vi "Actividad Extra 14 (2).vi"() -> ()   [LabVIEW 2018]
panel:
  out "Numeric 2":i32
  out "Pos Enemigos":i32
  out "Estado Actual":string
  out "Vidas Restantes":i32
  out "element 2":bool
  out "element 1":bool
  out "Posicion de la Nave":bool
  out "2":bool
  out "1":bool
  out "0":bool
  out "Disparos Restantes":i32
  out "Turno (5s)":i32 caption="Elapsed Time (s)"
  out "Nave Dispara Laser":bool
  in  "Disparar Laser":bool
  out "Nave Vuela a la Derecha":bool
  out "Nave Vuela a la Izq":bool
  in  "Izquierda":bool
  in  "Derecha":bool
  in  "ME RINDO":bool
  out "Jugador":bool[](array[boolean])
  out "Enemigos":bool[][](array[boolean])
  # "JUEGO NAVE ESPACIAL"
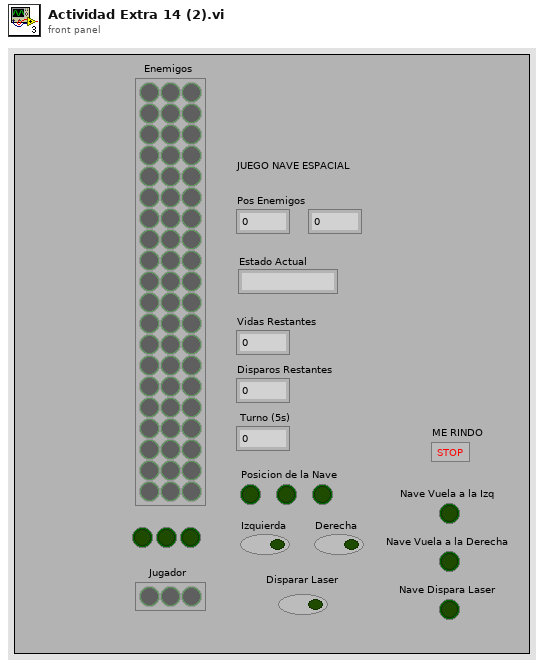
[diagram p1: front panel]
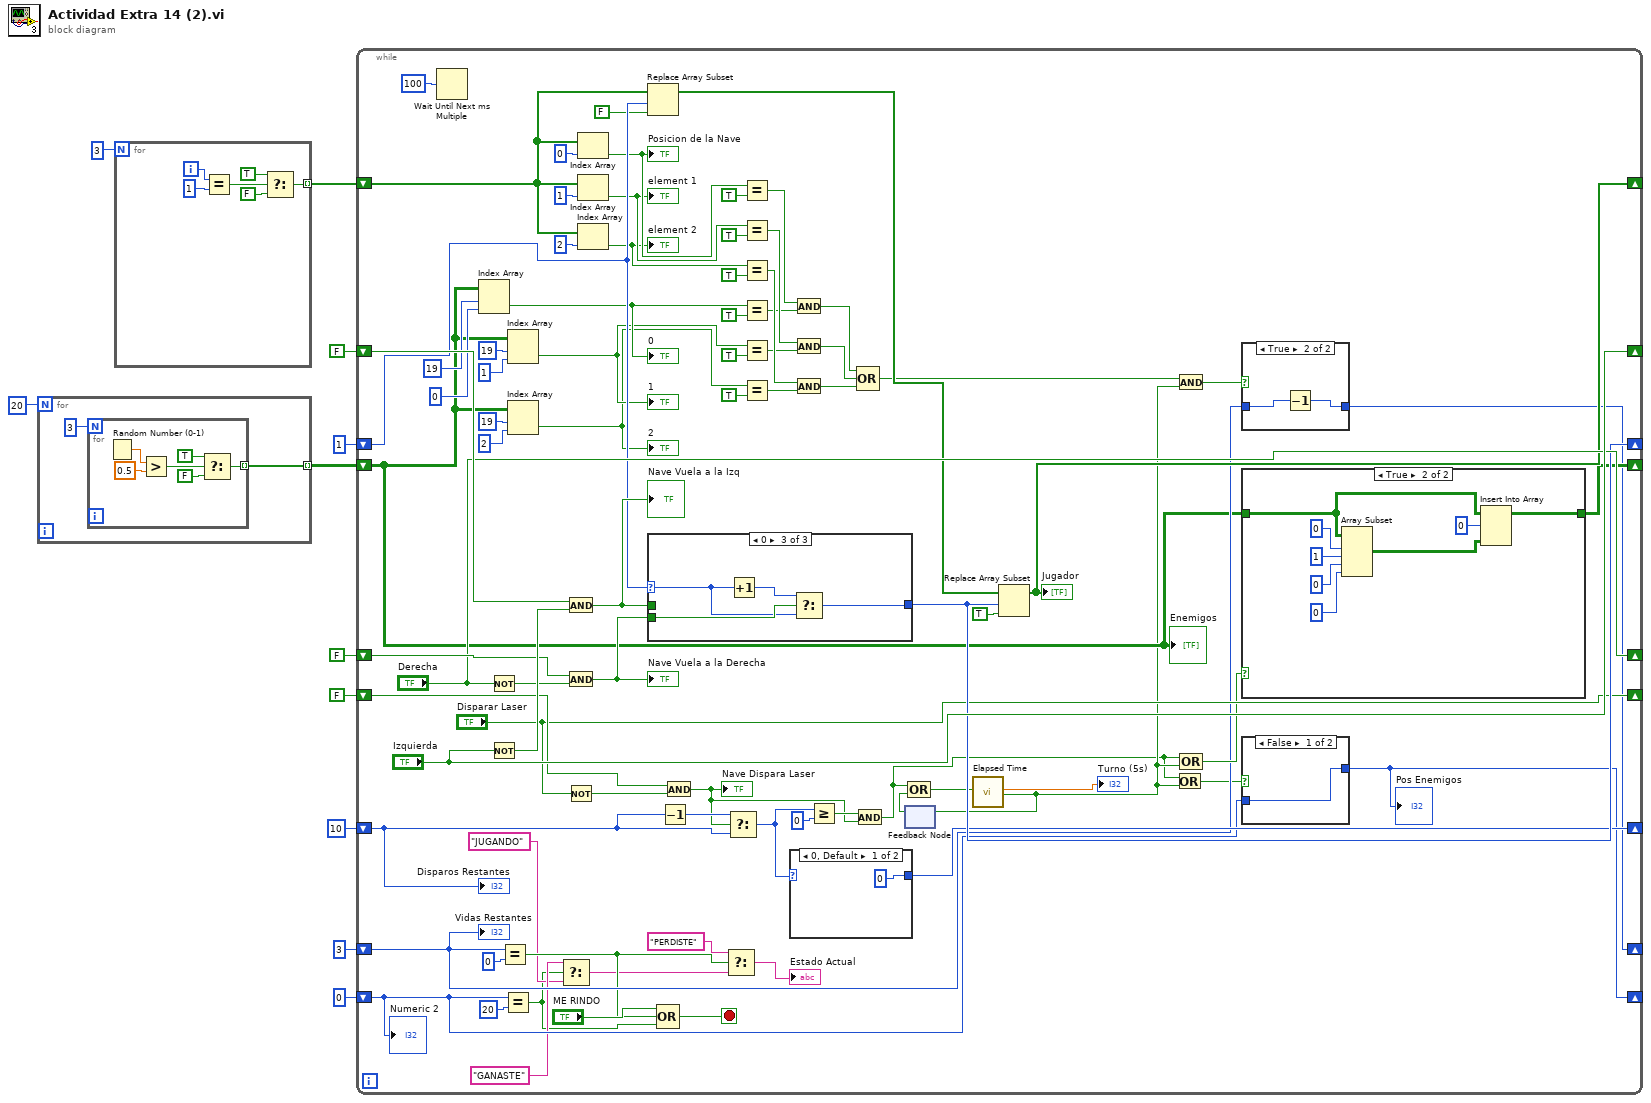
[diagram p0: block diagram]
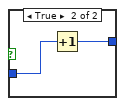
[diagram p2: hidden frame]
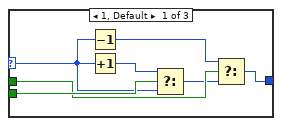
[diagram p6: hidden frame]
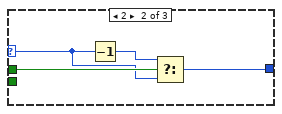
[diagram p7: hidden frame]
diagram:
  n1 = for {
    N: 20 -> [_]
    tunnel: [w12] -> w9 mode=indexing
    n2 = for {
      N: 3 -> [_]
      tunnel: [w14] -> w12 mode=indexing
      n3 = Random Number (0-1)() -> (number: 0 to 1=w19:dbl)
      n4 = Greater?(x=w19, y=0.5) -> (0:w17:bool)
      n5 = Select(t=TRUE, s=w17, f=FALSE) -> (s? t:f=w14:bool)
    }
  }
  n6 = for {
    N: 3 -> [_]
    tunnel: [w20] -> w8 mode=indexing
    i -> [w25]
    n7 = Equal?(x=w25, y=1) -> (x = y?=w23:bool)
    n8 = Select(t=TRUE, s=w23, f=FALSE) -> (s? t:f=w20:bool)
  }
  n9 = while {
    shift-right: [w93] -> _
    shift-left: w8 -> [w72]
    shift-right: [w89] -> _
    shift-left: w9 -> [w37]
    shift-right: ["Izquierda"] -> _
    shift-left: FALSE -> [w106]
    shift-right: ["Derecha"] -> _
    shift-left: FALSE -> [w103]
    shift-right: [w98] -> _
    shift-left: 1 -> [w97]
    shift-right: ["Disparar Laser"] -> _
    shift-left: FALSE -> [w92]
    shift-right: [w79] -> _
    shift-left: 10 -> [w84]
    shift-right: [w68] -> _
    shift-left: 3 -> [w67]
    shift-right: [w35] -> _
    shift-left: 0 -> [w31]
    stop <- w64 stop-if-true
    n10 = Wait Until Next ms Multiple(millisecond multiple=u32 100) -> ()  [unwired: 1 out]
    n11 = Index Array "Index Array"(array=w37, index (row)=19, index (col)=0 ("disabled index (col)")) -> (element=w44:bool)
    "0" <- w44
    n12 = Not(x="Derecha") -> (.not. x?=w102:bool)
    n13 = Not(x="Izquierda") -> (.not. x?=w105:bool)
    n14 = Equal?(x=w67, y=0) -> (x = y?=w40:bool)
    n15 = Equal?(x=w31, y=20) -> (x = y?=w26:bool)
    n16 = Index Array(array=w37, index (row)=19, index (col)=1 ("disabled index (col)")) -> (element=w43:bool)
    "1" <- w43
    n17 = Index Array(array=w37, index (row)=19, index (col)=2 ("disabled index (col)")) -> (element=w42:bool)
    "2" <- w42
    n18 = Select(t="GANASTE" ("f"), s=w26, f="JUGANDO") -> (s? t:f=w29:string)
    n19 = And(x=w106, y=w105) -> (x .and. y?=w99:bool)
    "Nave Vuela a la Izq" <- w99
    n20 = And(x=w103, y=w102) -> (x .and. y?=w100:bool)
    "Nave Vuela a la Derecha" <- w100
    n21 = Not(x="Disparar Laser") -> (.not. x?=w91:bool)
    n22 = Index Array(array=w72, index=0) -> (element=w62:bool)
    "Posicion de la Nave" <- w62
    n23 = Index Array(array=w72, index=1) -> (element=w60:bool)
    "element 1" <- w60
    n24 = Index Array(array=w72, index=2) -> (element=w57:bool)
    "element 2" <- w57
    n25 = Replace Array Subset "Replace Array Subset"(array=w72, new element=FALSE ("new element/subarray"), index=w97) -> (w95:bool[])
    n26 = case shown="0" w97 {
      selector: w97 -> [w127 w133 w136]
      tunnel: w100 -> [w131 _ w139]
      tunnel: [w125 w132 w137] -> w98
      tunnel: w99 -> [w129 w135 _]
      frame 1, Default {
        n27 = Decrement(x=w127) -> (x-1=w128:i32)
        n28 = Increment(x=w127) -> (x+1=w130:i32)
        n29 = Select(t=w130, s=w131, f=w127) -> (s? t:f=w126:i32)
        n30 = Select(t=w128, s=w129, f=w126) -> (s? t:f=w125:i32)
      }
      frame 2 {
        n31 = Decrement(x=w133) -> (x-1=w134:i32)
        n32 = Select(t=w134, s=w135, f=w133) -> (s? t:f=w132:i32)
      }
      frame 0 {
        n33 = Increment(x=w136) -> (x+1=w138:i32)
        n34 = Select(t=w138, s=w139, f=w136) -> (s? t:f=w137:i32)
      }
    }
    n35 = Compound Arithmetic op=OR("ME RINDO", w40, w26) -> (w64:bool)
    n36 = Decrement(x=w84) -> (x-1=w83:i32)
    n37 = And(x=w92, y=w91) -> (x .and. y?=w33:bool)
    "Nave Dispara Laser" <- w33
    n38 = Select(t="PERDISTE", s=w40, f=w29) -> (s? t:f=→"Estado Actual":string)
    n39 = Select(t=w83, s=w33, f=w84) -> (s? t:f=w80:i32)
    n40 = Equal?(x=w62, y=TRUE) -> (x = y?=w56:bool)
    n41 = Equal?(x=w60, y=TRUE) -> (x = y?=w55:bool)
    n42 = Equal?(x=w57, y=TRUE) -> (x = y?=w54:bool)
    n43 = Equal?(x=w44, y=TRUE) -> (x = y?=w48:bool)
    n44 = Equal?(x=w43, y=TRUE) -> (x = y?=w50:bool)
    n45 = Equal?(x=w42, y=TRUE) -> (x = y?=w49:bool)
    n46 = case shown="0, Default" w80 {
      selector: w80 -> [_ w115]
      tunnel: [0 w115] -> w79
      frame 0, Default {
      }
      frame 1.. {
      }
    }
    n47 = And(x=w56, y=w48) -> (x .and. y?=w47:bool)
    n48 = And(x=w55, y=w50) -> (x .and. y?=w46:bool)
    n49 = And(x=w54, y=w49) -> (x .and. y?=w45:bool)
    n50 = Greater Or Equal?(x=w80, y=0) -> (x >= y?=w81:bool)
    n51 = And(x=w81, y=w33) -> (x .and. y?=w30:bool)
    n52 = Compound Arithmetic op=OR(w47, w46, w45) -> (w41:bool)
    n53 = feedback #1() -> (w86:bool)  [unwired: 1 in]
    n54 = Compound Arithmetic op=OR(w30, w86) -> (w87:bool)
    n55 = call "Elapsed Time"("Reset"=w87) -> ("Elapsed Time (s)"=→"Turno (5s)":dbl, "Time has Elapsed"=w32:bool)  [unwired: 11 in, 6 out]
    n56 = feedback-in #1(w32) -> ()
    n57 = Replace Array Subset(array=w95, new element=TRUE ("new element/subarray"), index=w98) -> (w93:bool[])
    "Jugador" <- w93
    n58 = Or(x=w30, y=w32) -> (x .or. y?=w36:bool)
    n59 = And(x=w41, y=w32) -> (x .and. y?=w63:bool)
    n60 = Compound Arithmetic op=OR(w30, w32) -> (w85:bool)
    n61 = case shown="True" w63 {
      tunnel: w67 -> [w111 w113]
      tunnel: [w111 w112] -> w68
      frame False {
      }
      frame True {
        n62 = Decrement(x=w113) -> (x-1=w112:i32)
      }
    }
    n63 = case shown="True" w85 {
      tunnel: w37 -> [w116 w120]
      tunnel: [w116 w117] -> w89
      frame False {
      }
      frame True {
        n64 = Array Subset "Array Subset"(array=w120, index (row)=0 ("index"), length (row)=1 ("length"), index (col)=0 ("index"), length (col)=0 ("length")) -> (w119:bool[][])
        n65 = Insert Into Array "Insert Into Array"(array=w120, index (row)=0, new element=w119) -> (w117:bool[][])  [unwired: 1 in]
      }
    }
    n66 = case shown="False" w36 {
      tunnel: w31 -> [w108 w110]
      tunnel: [w108 w109] -> w35
      frame False {
      }
      frame True {
        n67 = Increment(x=w110) -> (x+1=w109:i32)
      }
    }
    "Pos Enemigos" <- w35
    "Enemigos" <- w37
    "Disparos Restantes" <- w84
    "Vidas Restantes" <- w67
    "Numeric 2" <- w31
  }
